vi "Main.vi"(10 "Communication":refnum<class "Communication.lvclass">, 11 "Module Admin":refnum<class "Delacor_lib_QMH_Cloneable Module Admin.lvclass">) -> ()   [LabVIEW 2021, in "Communication.lvlib"]
doc: "This template is based off of the Queued Message Handler design pattern and the Queued Message Handler project template that ships with LabVIEW.\n\nThe main difference is that the queue is private to this module and communication between modules is performed via Broadcast and Request events.\n\nRequest events are wrapped in public API methods and are handled in the Event Handling Loop (EHL) of this VI. Any module can register for Broadcast events sent by this module. The EHL generates messages based on user interface actions.\n\nThe Message Handling Loop (MHL) processes messages generated by the EHL, or by other messages. The messages are string values, so new messages can be added easily to the Message Cases case structure in the MHL. Each message cluster can also provide an optional value for Message Data, which is a variant that can be converted to whatever message-specific data is required.\n_____\nBased on DQMH Dev Tools: Project Template 7.1.2.1547."
uses:
  Communication.lvlib
  <vilib>/Delacor/Delacor QMH/Libraries/Cloneable Module Admin_class/Delacor_lib_QMH_Cloneable Module Admin.lvclass
  C:/Program Files (x86)/National Instruments/LabVIEW 2021/vi.lib/Delacor/Delacor QMH/Libraries/Module Admin_class/Delacor_lib_QMH_Module Admin.lvclass
  Communication/Communication.lvclass
  Module Data--cluster.ctl
  <vilib>/Delacor/Delacor QMH/Libraries/Message Queue_class/Delacor_lib_QMH_Message Queue.lvclass/Delacor_lib_QMH_Message Queue.ctl
  <vilib>/Delacor/Delacor QMH/Libraries/Cloneable Module Admin_class/Delacor_lib_QMH_Cloneable Module Admin.lvclass/Delacor_lib_QMH_Cloneable Module Admin.ctl
  Stop Argument--cluster.ctl
  <vilib>/Delacor/Delacor QMH/Libraries/Module Admin_class/Delacor_lib_QMH_Module Admin.lvclass/Delacor_lib_QMH_Module Admin.ctl
  Show config values Argument--cluster.ctl
  Show config values (Reply Payload)--cluster.ctl
  <vilib>/Utility/miscctls.llb/LVPointTypeDef.ctl
  Communication/Communication.lvclass/Communication.ctl
  <vilib>/Delacor/Delacor QMH/Libraries/Message Queue_class/Delacor_lib_QMH_Enqueue Message (Single).vi
  <vilib>/Delacor/Delacor QMH/Libraries/Cloneable Module Admin_class/Delacor_lib_QMH_Get Module ID.vi
  <vilib>/Delacor/Delacor QMH/Libraries/Module Admin_class/Delacor_lib_QMH_Get External Launch.vi
  <vilib>/Delacor/Delacor QMH/Libraries/Message Queue_class/Delacor_lib_QMH_Message Queue.lvclass
panel:
  out "error out":errorcluster
  out "Status":string
  in  "Simulate EHL Error":bool
  in  "Simulate MHL Error":bool
  # "Other processes communicate with this Module via its Public API (wrappers for its Request Events).\n\nThis Module communicates with other processes via its Broadcast Events.\nAny process that wants to receive these messages can register for this module's Broadcast events."
  # "This template is for the DQMH framework. See the block diagram for more information on how to use this template."
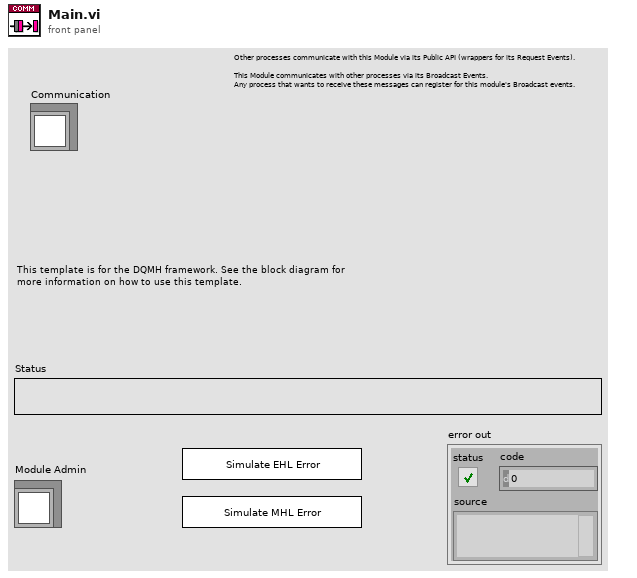
[diagram p1: front panel]
types:
  T1 = typedef "Communication.lvlib/Request Events--cluster.ctl" = cluster{"Stop Module":refnum<user-event>, "Show Panel":refnum<user-event>, "Hide Panel":refnum<user-event>, "Show Diagram":refnum<user-event>, "Get Module Execution Status":refnum<user-event>, "Show config values":refnum<user-event>}
  T2 = typedef "Communication.lvlib/Module Data--cluster.ctl" = cluster{"Status":string}
  T3 = enum32{"invalid lock state", "Not Locked", "Locked (No Password)", "Password-protected"}
  T4 = typedef "Communication.lvlib/Stop Argument--cluster.ctl" = cluster{"Module ID":i32, "Origin":string, "Exit via Stop Module Req?":bool, "Wait for Module to stop?":bool}
  T5 = typedef "Communication.lvlib/Show config values Argument--cluster.ctl" = cluster{"Module ID":i32, "Wait Notifier":refnum<notifier>, "wait for reply":bool}
  T6 = typedef "LVPointTypeDef.ctl" = cluster{"Horizontal":i16, "Vertical":i16}
  T7 = enum32{"Invalid", "Standard", "Closed", "Hidden", "Minimized", "Maximized"}
  T8 = typedef "Communication.lvlib/Show config values (Reply Payload)--cluster.ctl" = cluster{"Module ID":i32, "Comm":cluster{"Path":path}, "error":errorcluster, "params":cluster{"connection_type":string, "baud_rate":i32, "port":string, "Name":string, "ShowFP":bool}}
  T9 = cluster{"connection_type":string, "baud_rate":i32, "port":string, "Name":string, "ShowFP":bool}
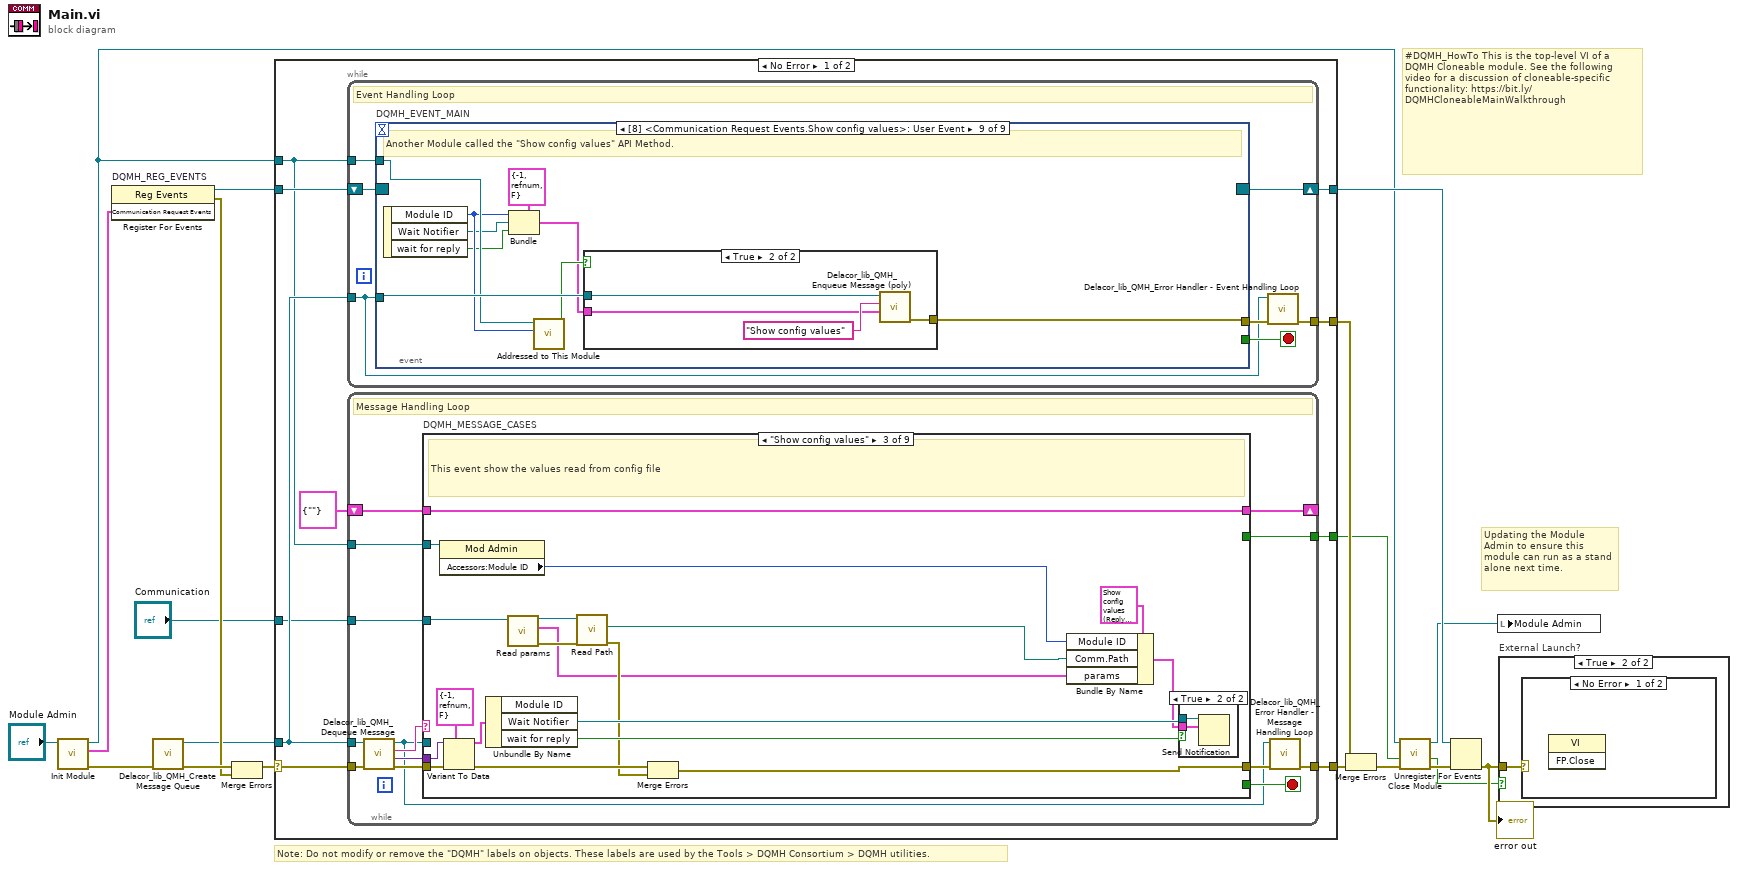
[diagram p0: block diagram]
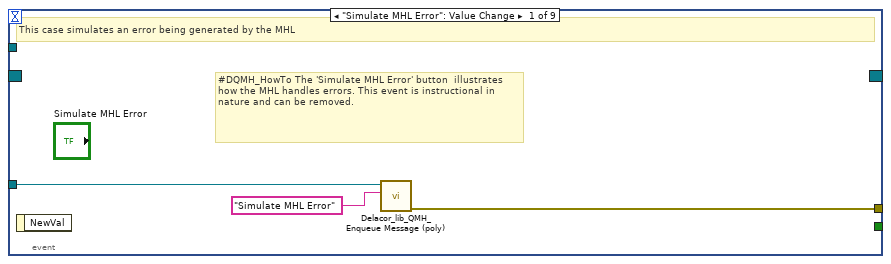
[diagram p2: hidden frame]
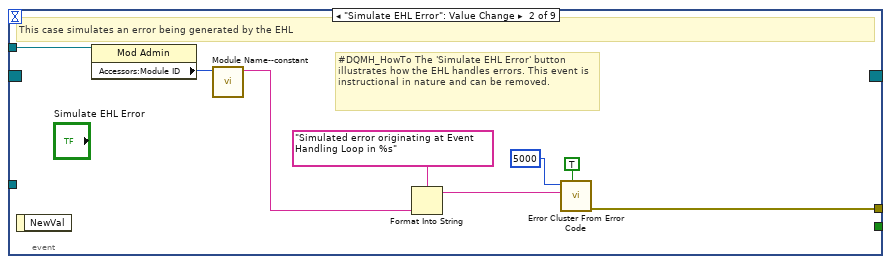
[diagram p3: hidden frame]
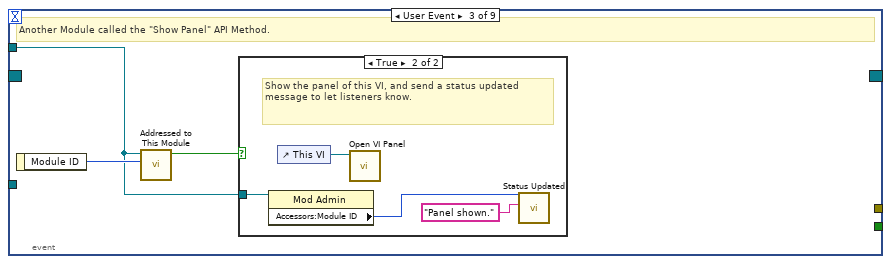
[diagram p4: hidden frame]
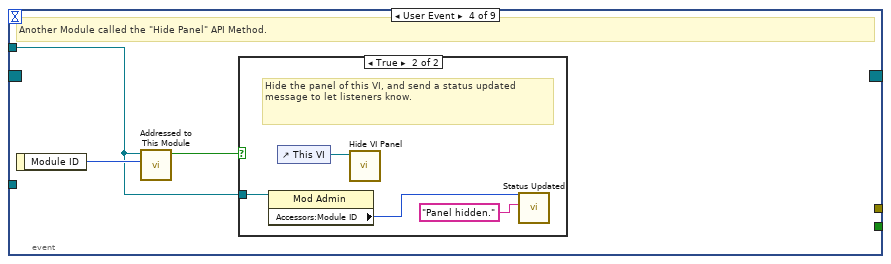
[diagram p6: hidden frame]
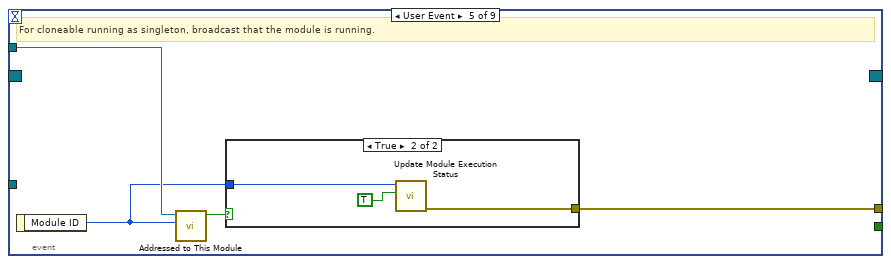
[diagram p8: hidden frame]
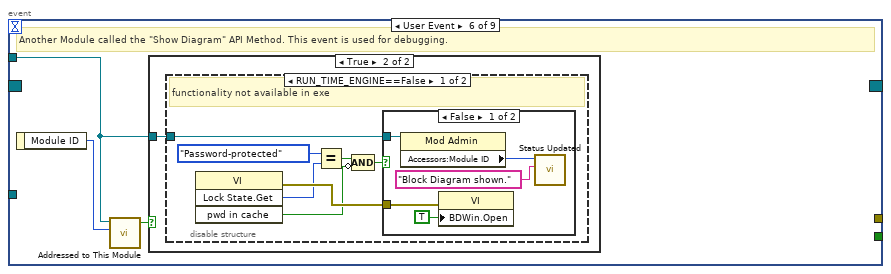
[diagram p10: hidden frame]
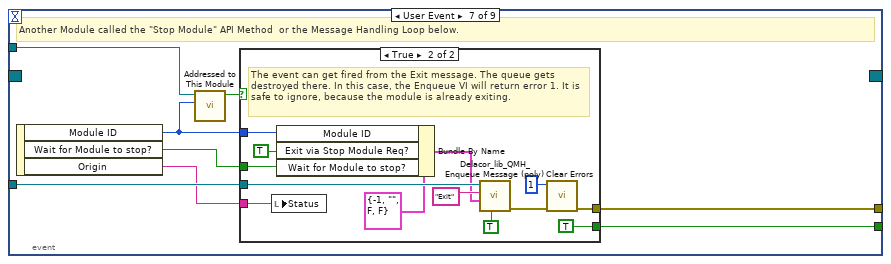
[diagram p14: hidden frame]
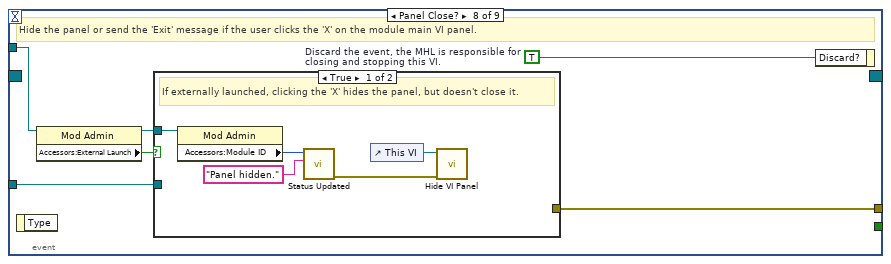
[diagram p16: hidden frame]
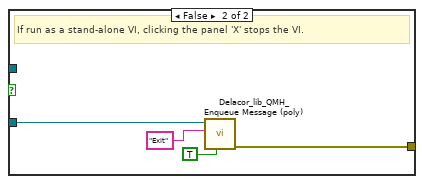
[diagram p17: hidden frame]
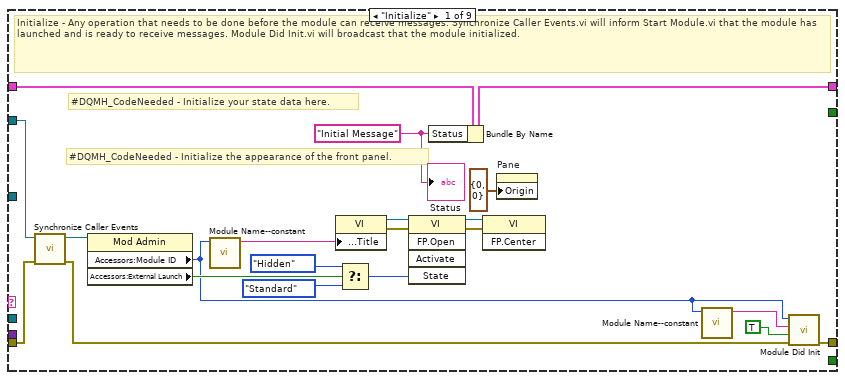
[diagram p19: hidden frame]
diagram:
  # "#DQMH_HowTo This is the top-level VI of a DQMH Cloneable module. See the following video for a discussion of cloneable-specific functionality: https://bit.ly/DQMHCloneableMainWalkthrough"
  # "Note: Do not modify or remove the \"DQMH\" labels on objects. These labels are used by the Tools > DQMH Consortium > DQMH utilities."
  # "Updating the Module Admin to ensure this module can run as a stand alone next time."
  n1 = call "Init Module.vi"("Cloneable Module Admin in"="Module Admin") -> ("error out"=w16:errorcluster, "Communication Request Events"=w8:T1, "Cloneable Module Admin out"=w5:refnum<class "Delacor_lib_QMH_Cloneable Module Admin.lvclass">)  [unwired: 8 in]
  n2 = register-events "DQMH_REG_EVENTS"(w8) -> (reference out=w9:refnum<event-registration>, error out=w11:errorcluster)  [unwired: 2 in]
  n3 = call <vilib>:"Delacor_lib_QMH_Create Message Queue.vi"("error in"=w16) -> ("error out"=w13:errorcluster, "Message Queue"=w7:refnum<class "Delacor_lib_QMH_Message Queue.lvclass">)  [unwired: 9 in]
  n4 = Merge Errors(w13, w11) -> (w12:errorcluster)
  n5 = case shown="No Error" w12 {
    selector: w12 -> [w27 w264]
    tunnel: [w29 w263] -> w17
    tunnel: [w26 w262] -> w10
    tunnel: w9 -> [w24 w262]
    tunnel: w7 -> [w23 w255]
    tunnel: [w28 _] -> w18
    tunnel: w5 -> [w22 w258]
    tunnel: [w21 _] -> w3
    tunnel: "Communication" -> [w20 _]
    frame No Error {
      n6 = while {
        tunnel: w23 -> [w30]
        shift-right: [w33] -> w26
        shift-left: w24 -> [w34]
        tunnel: [w35] -> w28
        tunnel: w22 -> [w31]
        stop <- w32 stop-if-true
        # "Event Handling Loop"
        n7 = event "DQMH_EVENT_MAIN" shown="[8] <Communication Request Events.Show config values>: User Event" {
          selector: w34 -> [_ _ _ _ _ _ _ _ _]
          dyn-events: [_ _ _ _ _ _ _ _ _] -> w33
          timeout: _ -> [_ _ _ _ _ _ _ _ _]
          tunnel: [_ _ _ _ _ _ w88 _ _] -> w32
          tunnel: w30 -> [w38 _ _ _ _ _ w91 w108 w129]
          tunnel: [w39 w47 _ _ w65 _ w92 w111 w121] -> w36
          tunnel: w31 -> [_ w46 w48 w55 w63 w69 w90 w109 w127]
          event "Simulate MHL Error": Value Change {
            # "#DQMH_HowTo The 'Simulate MHL Error' button  illustrates how the MHL handles errors. This event is instructional in nature and can be removed."
            # "This case simulates an error being generated by the MHL"
            n8 = event-data() -> ()  [unwired: 1 in, 1 out]
            n9 = call-poly <vilib>:"Delacor_lib_QMH_Enqueue Message (poly).vi"("Message"="Simulate MHL Error", "Message Queue in"=w38) -> ("error out"=w39:errorcluster)  [unwired: 8 in, 1 out]
          }
          event "Simulate EHL Error": Value Change {
            # "#DQMH_HowTo The 'Simulate EHL Error' button  illustrates how the EHL handles errors. This event is instructional in nature and can be removed."
            # "This case simulates an error being generated by the EHL"
            n10 = event-data() -> ()  [unwired: 1 in, 1 out]
            n11 = property on="Property Node" class="Mod Admin"(reference=w46) -> ("Accessors:Module ID"=w45:i32)  [unwired: 1 in, 2 out]
            n12 = call "Module Name--constant.vi"("Module ID"=w45) -> ("Module Name"=w40:string)  [unwired: 10 in]
            n13 = Format Into String(format string="Simulated error originating at Event Handling Loop in %s", w40) -> (resulting string=w43:string)  [unwired: 2 in, 1 out]
            n14 = call <vilib>:"Error Cluster From Error Code.vi"("show call chain? (False)"=TRUE, "error message (\"\")"=w43, "error code (0)"=5000) -> ("error out"=w47:errorcluster)  [unwired: 6 in]
          }
          event User Event {
            # "Another Module called the \"Show Panel\" API Method."
            n15 = event-data() -> ("Module ID"=w49:i32)  [unwired: 1 in]
            n16 = call "Addressed to This Module.vi"("Module ID from Argument"=w49, "Module Admin"=w48) -> ("Addressed to this instance?"=w50:bool)  [unwired: 8 in, 1 out]
            n17 = case shown="True" w50 {
              tunnel: w48 -> [_ w52]
              frame False {
              }
              frame True {
                # "Show the panel of this VI, and send a status updated message to let listeners know."
                n18 = property on="Property Node" class="Mod Admin"(reference=w52) -> ("Accessors:Module ID"=w51:i32)  [unwired: 1 in, 2 out]
                n19 = control-ref of="This VI"() -> (w54:refnum<vi>)
                n20 = call "Open VI Panel.vi"("VI"=w54) -> ()  [unwired: 10 in, 1 out]
                n21 = call "Status Updated.vi"("Status"="Panel shown." ("format string"), "Module ID"=w51) -> ()  [unwired: 9 in, 1 out]
              }
            }
          }
          event User Event {
            # "Another Module called the \"Hide Panel\" API Method."
            n22 = event-data() -> ("Module ID"=w56:i32)  [unwired: 1 in]
            n23 = call "Addressed to This Module.vi"("Module ID from Argument"=w56, "Module Admin"=w55) -> ("Addressed to this instance?"=w57:bool)  [unwired: 8 in, 1 out]
            n24 = case shown="True" w57 {
              tunnel: w55 -> [_ w59]
              frame False {
              }
              frame True {
                # "Hide the panel of this VI, and send a status updated message to let listeners know."
                n25 = property on="Property Node" class="Mod Admin"(reference=w59) -> ("Accessors:Module ID"=w58:i32)  [unwired: 1 in, 2 out]
                n26 = control-ref of="This VI"() -> (w61:refnum<vi>)
                n27 = call "Hide VI Panel.vi"("VI"=w61) -> ()  [unwired: 10 in, 1 out]
                n28 = call "Status Updated.vi"("Status"="Panel hidden." ("format string"), "Module ID"=w58) -> ()  [unwired: 9 in, 1 out]
              }
            }
          }
          event User Event {
            # "For cloneable running as singleton, broadcast that the module is running."
            n29 = event-data() -> ("Module ID"=w62:i32)  [unwired: 1 in]
            n30 = call "Addressed to This Module.vi"("Module ID from Argument"=w62, "Module Admin"=w63) -> ("Addressed to this instance?"=w64:bool)  [unwired: 8 in, 1 out]
            n31 = case shown="True" w64 {
              tunnel: [_ w68] -> w65
              tunnel: w62 -> [_ w67]
              frame False {
              }
              frame True {
                n32 = call "Update Module Execution Status.vi"("Running?"=TRUE, "Module ID"=w67) -> ("error out"=w68:errorcluster)  [unwired: 9 in]
              }
            }
          }
          event User Event {
            # "Another Module called the \"Show Diagram\" API Method. This event is used for debugging."
            n33 = event-data() -> ("Module ID"=w70:i32)  [unwired: 1 in]
            n34 = call "Addressed to This Module.vi"("Module ID from Argument"=w70, "Module Admin"=w69) -> ("Addressed to this instance?"=w71:bool)  [unwired: 8 in, 1 out]
            n35 = case shown="True" w71 {
              tunnel: w69 -> [_ w72]
              frame False {
              }
              frame True {
                n36 = disable-structure shown="RUN_TIME_ENGINE==False" {
                  disable-tunnel: w72 -> [w73 _]
                  frame condition #0 (active) {
                    # "functionality not available in exe"
                    n37 = invoke on="Invoke Node" class="VI" method="Lock State.Get"() -> (error out=w79:errorcluster, "Get Lock State"=w78:T3, "pwd in cache"=w75:bool)  [unwired: 4 in, 1 out]
                    n38 = Equal?(x=T3."Password-protected", y=w78) -> (x = y?=w76:bool)
                    n39 = Compound Arithmetic op=AND(w76, invert w75) -> (w74:bool)
                    n40 = case shown="False" w74 {
                      tunnel: w79 -> [w84 _]
                      tunnel: w73 -> [w81 _]
                      frame False {
                        n41 = property on="Property Node" class="Mod Admin"(reference=w81) -> ("Accessors:Module ID"=w80:i32)  [unwired: 1 in, 2 out]
                        n42 = property on="Property Node" class="VI"(error in=w84, "BDWin.Open"=TRUE ("Block Diagram Window:Open")) -> ()  [unwired: 1 in, 2 out]
                        n43 = call "Status Updated.vi"("Status"="Block Diagram shown." ("format string"), "Module ID"=w80) -> ()  [unwired: 9 in, 1 out]
                      }
                      frame True {
                        # "Password-protected VI, and the password is not in the cache. Do not show the diagram."
                      }
                    }
                  }
                  frame condition #1 {
                  }
                }
              }
            }
          }
          event User Event {
            # "Another Module called the \"Stop Module\" API Method  or the Message Handling Loop below."
            n44 = event-data() -> ("Module ID"=w86:i32, "Wait for Module to stop?"=w87:bool, "Origin"=w85:string)  [unwired: 1 in]
            n45 = call "Addressed to This Module.vi"("Module ID from Argument"=w86, "Module Admin"=w90) -> ("Addressed to this instance?"=w89:bool)  [unwired: 8 in, 1 out]
            n46 = case shown="True" w89 {
              tunnel: [_ w104] -> w92
              tunnel: w91 -> [_ w100]
              tunnel: [_ TRUE] -> w88
              tunnel: w87 -> [_ w95]
              tunnel: w86 -> [_ w97]
              tunnel: w85 -> [_ w93]
              frame False {
              }
              frame True {
                # "The event can get fired from the Exit message. The queue gets destroyed there. In this case, the Enqueue VI will return error 1. It is safe to ignore, because the module is already exiting."
                n47 = local write "Status"(w93) -> ()
                n48 = Bundle By Name(cluster=T4 {"Module ID"=-1, "Origin"="", "Exit via Stop Module Req?"=FALSE, "Wait for Module to stop?"=FALSE} ("Stop Argument"), "Module ID"=w97, "Exit via Stop Module Req?"=TRUE, "Wait for Module to stop?"=w95) -> (w94:T4)
                n49 = call-poly <vilib>:"Delacor_lib_QMH_Enqueue Message (poly).vi"("Priority Message? (F)"=TRUE, "Message Data"=w94, "Message"="Exit", "Message Queue in"=w100) -> ("error out"=w105:errorcluster)  [unwired: 6 in, 1 out]
                n50 = call <vilib>:"Clear Errors.vi"("error in (no error)"=w105, "specific error code to clear (0: all)"=1) -> ("error out"=w104:errorcluster)  [unwired: 4 in, 1 out]
              }
            }
          }
          event Panel Close? {
            w110 = TRUE  # Discard the event, the MHL is responsible for closing and stopping this VI.
            # "Hide the panel or send the 'Exit' message if the user clicks the 'X' on the module main VI panel."
            n51 = event-data() -> ()  [unwired: 1 in, 1 out]
            n52 = property on="Property Node" class="Mod Admin"(reference=w109) -> (reference out=w106:refnum<class "Delacor_lib_QMH_Cloneable Module Admin.lvclass">, "Accessors:External Launch"=w107:bool)  [unwired: 1 in, 1 out]
            n53 = case shown="True" w107 {
              tunnel: w108 -> [_ w119]
              tunnel: [_ w120] -> w111
              tunnel: w106 -> [w114 _]
              frame True {
                # "If externally launched, clicking the 'X' hides the panel, but doesn't close it."
                n54 = property on="Property Node" class="Mod Admin"(reference=w114) -> ("Accessors:Module ID"=w113:i32)  [unwired: 1 in, 2 out]
                n55 = call "Status Updated.vi"("Status"="Panel hidden." ("format string"), "Module ID"=w113) -> ("error out"=w112:errorcluster)  [unwired: 9 in]
                n56 = control-ref of="This VI"() -> (w116:refnum<vi>)
                n57 = call "Hide VI Panel.vi"("error in"=w112, "VI"=w116) -> ()  [unwired: 9 in, 1 out]
              }
              frame False {
                # "If run as a stand-alone VI, clicking the panel 'X' stops the VI."
                n58 = call-poly <vilib>:"Delacor_lib_QMH_Enqueue Message (poly).vi"("Priority Message? (F)"=TRUE, "Message"="Exit", "Message Queue in"=w119) -> ("error out"=w120:errorcluster)  [unwired: 7 in, 1 out]
              }
            }
            n59 = event-data ("Event Filter Node")("Discard?"=w110) -> ()  [unwired: 1 in, 1 out]
          }
          event User Event {
            # "Another Module called the \"Show config values\" API Method."
            n60 = event-data() -> ("Module ID"=w124:i32, "Wait Notifier"=w123:refnum<notifier>, "wait for reply"=w122:bool)  [unwired: 1 in]
            n61 = Bundle(cluster=T5 {"Module ID"=-1, "Wait Notifier"=refnum, "wait for reply"=FALSE} ("Show config values Argument"), "Module ID"=w124, "Wait Notifier"=w123, "wait for reply"=w122) -> (w125:T5)
            n62 = call "Addressed to This Module.vi"("Module ID from Argument"=w124, "Module Admin"=w127) -> ("Addressed to this instance?"=w128:bool)  [unwired: 8 in, 1 out]
            n63 = case shown="True" w128 {
              tunnel: w129 -> [_ w133]
              tunnel: w125 -> [_ w131]
              tunnel: [_ w130] -> w121
              frame False {
              }
              frame True {
                n64 = call-poly <vilib>:"Delacor_lib_QMH_Enqueue Message (poly).vi"("Message Data"=w131, "Message"="Show config values", "Message Queue in"=w133) -> ("error out"=w130:errorcluster)  [unwired: 7 in, 1 out]
              }
            }
          }
        }
        n65 = call-dynamic "Delacor_lib_QMH_Error Handler - Event Handling Loop.vi"("error in"=w36, "Message Queue in"=w30) -> ("dup error in"=w35:errorcluster)  [unwired: 8 in, 1 out]
      }
      n66 = while {
        tunnel: w23 -> [w135]
        shift-right: [w142] -> _
        shift-left: T2 {"Status"=""} ("Data Cluster") -> [w143]
        tunnel: w27 -> [w146]
        tunnel: [w144] -> w29
        tunnel: w22 -> [w137]
        tunnel: [w136] -> w21
        tunnel: w20 -> [w134]
        stop <- w141 stop-if-true
        # "Message Handling Loop"
        n67 = call-dynamic "Delacor_lib_QMH_Dequeue Message.vi"("error in"=w146, "Message Queue in"=w135) -> ("error out"=w145:errorcluster, "Message Data"=w139:variant, "Message"=w140:string, "Message Queue out"=w138:refnum<class "Delacor_lib_QMH_Message Queue.lvclass">)  [unwired: 6 in]
        n68 = case "DQMH_MESSAGE_CASES" shown="\"Show config values\"" w140 {
          selector: w140 -> [_ _ _ _ _ _ _ _ w244]
          tunnel: w138 -> [_ _ _ _ _ w199 _ w236 _]
          tunnel: w145 -> [w166 w170 w189 w194 w196 w208 w225 w242 w253]
          tunnel: [w164 w170 w179 w193 w196 w204 w224 w237 w254] -> w147
          tunnel: w143 -> [w157 w169 w188 w192 w195 w203 w222 w235 w251]
          tunnel: [w156 w169 w188 w192 w195 w203 w222 w235 w251] -> w142
          tunnel: [_ _ _ _ _ _ _ w234 _] -> w141
          tunnel: w139 -> [_ _ w186 _ _ w202 _ w232 _]
          tunnel: w137 -> [w152 _ w177 _ _ w201 w220 w227 w250]
          tunnel: [_ _ _ _ _ _ _ w230 _] -> w136
          tunnel: w134 -> [_ _ w173 _ _ _ _ _ _]
          frame "Initialize" {
            w149 = "Initial Message" ("Initial Message")
            # "#DQMH_CodeNeeded - Initialize the appearance of the front panel."
            # "#DQMH_CodeNeeded - Initialize your state data here."
            # "Initialize - Any operation that needs to be done before the module can receive messages. Synchronize Caller Events.vi will inform Start Module.vi that the module has launched and is ready to receive messages. Module Did Init.vi will broadcast that the module initialized."
            n69 = call "Synchronize Caller Events.vi"("error in"=w166, "Module Admin"=w152) -> ("error out"=w165:errorcluster, "Module Admin out"=w151:refnum<class "Delacor_lib_QMH_Cloneable Module Admin.lvclass">)  [unwired: 8 in]
            n70 = property on="Property Node" class="Mod Admin"(reference=w151) -> ("Accessors:Module ID"=w148:i32, "Accessors:External Launch"=w153:bool)  [unwired: 1 in, 2 out]
            n71 = call "Module Name--constant.vi"("Module ID"=w148) -> ("Module Name"=w161:string)  [unwired: 10 in]
            n72 = property on="Property Node" class="VI"("Front Panel.Title"=w161) -> (reference out=w163:refnum<vi>, error out=w168:errorcluster)  [unwired: 2 in]
            n73 = Select(t=T7."Hidden" ("State"), s=w153, f=T7."Standard" ("State")) -> (s? t:f=w158:T7)
            n74 = invoke on="Invoke Node" class="VI" method="FP.Open"(reference=w163, error in=w168, "State"=w158) -> (reference out=w162:refnum<vi>, error out=w167:errorcluster)  [unwired: 2 in, 3 out]
            n75 = Bundle By Name(cluster=w157, "Status"=w149) -> (w156:T2)
            n76 = invoke on="Invoke Node" class="VI" method="FP.Center"(reference=w162, error in=w167) -> ()  [unwired: 1 in, 3 out]
            n77 = property on="Pane" class="Pane"("Origin"=T6 {"Horizontal"=0, "Vertical"=0}) -> ()  [unwired: 2 in, 2 out]
            n78 = call "Module Name--constant.vi"("Module ID"=w148) -> ("Module Name"=w154:string)  [unwired: 10 in]
            n79 = call "Module Did Init.vi"("error in"=w165, "Initialized?"=TRUE, "Origin"=w154, "Module ID"=w148) -> ("error out"=w164:errorcluster)  [unwired: 7 in]
            "Status" <- w149
          }
          frame "---Module Specific---" {
            # "Separator -- The following cases handle messages specific to this Module."
          }
          frame "Show config values" {
            # "This event show the values read from config file"
            n80 = property class="Mod Admin"(reference=w177) -> ("Accessors:Module ID"=w178:i32)  [unwired: 1 in, 2 out]
            n81 = Variant To Data(error in=w189, type=T5 {"Module ID"=-1, "Wait Notifier"=refnum, "wait for reply"=FALSE} ("Show config values Argument"), Variant=w186) -> (data=w184:T5, error out=w187:errorcluster)
            n82 = Unbundle By Name(w184) -> ("Wait Notifier"=w183:refnum<notifier>, "wait for reply"=w182:bool)  [unwired: 1 out]
            n83 = call "Read params.vi"("Communication in"=w173) -> ("error out"=w174:errorcluster, "params"=w171:T9, "Communication out"=w175:refnum<class "Communication.lvclass">)  [unwired: 8 in]
            n84 = call "Read Path.vi"("error in (no error)"=w174, "Communication in"=w175) -> ("error out"=w172:errorcluster, "Path"=w176:path)  [unwired: 7 in, 1 out]
            n85 = Merge Errors(w187, w172) -> (w179:errorcluster)
            n86 = Bundle By Name(cluster=T8 {"Module ID"=-1, "Comm"={"Path"=path ""}, "error"={"status"=FALSE, "code"=0, "source"=""}, "params"={"connection_type"="", "baud_rate"=0, "port"="", "Name"="", "ShowFP"=FALSE}} ("Show config values (Reply Payload)"), "Module ID"=w178, "Comm.Path"=w176, "params"=w171) -> (w181:T8)
            n87 = case "DQMH_FIRE_NOTIFIER" shown="True" w182 {
              tunnel: w183 -> [_ w191]
              tunnel: w181 -> [_ w190]
              frame False {
              }
              frame True {
                n88 = Send Notification(notification=w190, notifier=w191) -> ()  [unwired: 1 in, 2 out]
              }
            }
          }
          frame "---Copy This Frame---" {
            # "Duplicate this frame when creating new messages.  Change this comment in the duplicated frame to describe this message."
            n89 = Merge Errors(w194) -> (w193:errorcluster)
          }
          frame "---Exit and Error Handling---" {
            # "Separator - the following cases handle errors and exit messages."
          }
          frame "Error" {
            # "#DQMH_CodeRecommended - If the module is running in standalone mode (External Launch = FALSE), this code will pop up an error dialog and call the 'Exit' message if an error occurs. Add more fine-grained error management here."
            # "Error - Check the error message data and respond accordingly. This message is sent by the \"Error Handler\" VIs at the end of each loop in this application."
            n90 = property on="Property Node" class="Mod Admin"(reference=w201) -> ("Accessors:External Launch"=w200:bool, "Accessors:Module ID"=w198:i32)  [unwired: 1 in, 2 out]
            n91 = Variant To Data(error in=w208, type=errorcluster {"status"=FALSE, "code"=0, "source"=""} ("error constant"), Variant=w202) -> (data=w197:errorcluster, error out=w206:errorcluster)
            n92 = local write "error out"(w197) -> ()
            n93 = call "Error Reported.vi"("Error"=w197, "Module ID"=w198) -> ()  [unwired: 9 in, 1 out]
            n94 = case shown="False" w200 {
              tunnel: [w213 _] -> w205
              tunnel: w199 -> [w211 _]
              tunnel: w197 -> [w212 _]
              frame False {
                n95 = disable-structure shown="Default" {
                  disable-tunnel: w212 -> [w214 _]
                  frame condition #0 (active) {
                    # "If the module is running standalone, then pop up an error dialog and call the \"Exit\" message."
                    n96 = call <vilib>:"Simple Error Handler.vi"("error in (no error)"=w214) -> ()  [unwired: 4 in, 5 out]
                  }
                  frame condition #1 {
                    # "To prevent the Simple Error Handler VI from being loaded (e.g. when deploying to a Real-Time target), add the Conditional Disable Symbol \"DQMH_Disable_SEH\" to your project and set it to TRUE."
                  }
                }
                n97 = call-poly <vilib>:"Delacor_lib_QMH_Enqueue Message (poly).vi"("Priority Message? (F)"=TRUE, "Message"="Exit", "Message Queue in"=w211) -> ("error out"=w213:errorcluster)  [unwired: 7 in, 1 out]
              }
              frame True {
                # "If the module was launched externally, calling the Error Reported broadcast VI is the only action performed by the \"Error\" message. The module's caller can then process the error appropriately."
              }
            }
            n98 = Merge Errors(w206, w205) -> (w204:errorcluster)
          }
          frame "Simulate MHL Error" {
            # "#DQMH_HowTo The 'Simulate MHL Error' button  illustrates how the MHL handles errors. This event is instructional in nature and can be removed."
            # "Simulate an error occurring at the MHL"
            n99 = property on="Property Node" class="Mod Admin"(reference=w220) -> ("Accessors:Module ID"=w221:i32)  [unwired: 1 in, 2 out]
            n100 = call "Module Name--constant.vi"("Module ID"=w221) -> ("Module Name"=w216:string)  [unwired: 10 in]
            n101 = Format Into String(format string="Simulated error originating at Message Handling Loop in %s", w216) -> (resulting string=w217:string)  [unwired: 2 in, 1 out]
            n102 = call <vilib>:"Error Cluster From Error Code.vi"("show call chain? (False)"=TRUE, "error message (\"\")"=w217, "error code (0)"=5001) -> ("error out"=w223:errorcluster)  [unwired: 6 in]
            n103 = Merge Errors(w225, w223) -> (w224:errorcluster)
          }
          frame "Exit" {
            w233 = 91  # 91: not all Exit messages will have an argument
            w234 = TRUE  # Stop the VI
            # "Release the message queue reference"
            # "#DQMH_CodeNeeded - Add any required cleanup code here."
            # "Exit - Exit the application."
            n104 = Variant To Data(error in=w242, type=T4 {"Module ID"=-1, "Origin"="", "Exit via Stop Module Req?"=FALSE, "Wait for Module to stop?"=FALSE} ("Stop Argument"), Variant=w232) -> (data=w229:T4, error out=w238:errorcluster)
            n105 = call <vilib>:"Clear Errors.vi"("error in (no error)"=w238, "specific error code to clear (0: all)"=w233) -> ("error out"=w241:errorcluster)  [unwired: 4 in, 1 out]
            n106 = property on="Property Node" class="Mod Admin"(reference=w227) -> ("Accessors:Module ID"=w226:i32)  [unwired: 1 in, 2 out]
            n107 = control-ref of="This VI"() -> (w228:refnum<vi>)
            n108 = call-dynamic "Delacor_lib_QMH_Release Message Queue.vi"("error in"=w241, "Message Queue"=w236) -> ("error out"=w240:errorcluster)  [unwired: 9 in]
            n109 = call "Handle Exit.vi"("Stop Argument"=w229, "Module Admin in"=w227, "VI reference"=w228) -> ("error out"=w239:errorcluster, "Wait for Stop?"=w230:bool)  [unwired: 7 in]
            n110 = Merge Errors(w240, w239) -> (w237:errorcluster)
            n111 = call "Error Reported.vi"("Error"=w237, "Module ID"=w226) -> ()  [unwired: 9 in, 1 out]
          }
          frame Default {
            # "'Default' case only runs if there is a message that isn't defined in any of the other cases.  Output a programming error."
            n112 = property on="Property Node" class="Mod Admin"(reference=w250) -> ("Accessors:Module ID"=w249:i32)  [unwired: 1 in, 2 out]
            n113 = call "Module Name--constant.vi"("Module ID"=w249) -> ("Module Name"=w243:string)  [unwired: 10 in]
            n114 = Format Into String(format string="The invalid message string \"%s\" was received in the Message Handling Loop for module \"%s\".", w244, w243) -> (resulting string=w246:string)  [unwired: 2 in, 1 out]
            n115 = call <vilib>:"Error Cluster From Error Code.vi"("show call chain? (False)"=TRUE, "error message (\"\")"=w246, "error code (0)"=1) -> ("error out"=w252:errorcluster)  [unwired: 6 in]
            n116 = Merge Errors(w253, w252) -> (w254:errorcluster)
          }
        }
        n117 = call-dynamic "Delacor_lib_QMH_Error Handler - Message Handling Loop.vi"("error in"=w147, "Message Queue in"=w138) -> ("dup error in"=w144:errorcluster)  [unwired: 8 in, 1 out]
      }
    }
    frame Error {
      n118 = call "Synchronize Caller Events.vi"("Module Admin"=w258) -> ("Module Admin out"=w257:refnum<class "Delacor_lib_QMH_Cloneable Module Admin.lvclass">)  [unwired: 9 in, 1 out]
      n119 = property on="Property Node" class="Mod Admin"(reference=w257) -> ("Accessors:Module ID"=w256:i32)  [unwired: 1 in, 2 out]
      n120 = call-dynamic "Delacor_lib_QMH_Release Message Queue.vi"("error in"=w264, "Message Queue"=w255) -> ("error out"=w263:errorcluster)  [unwired: 9 in]
      n121 = call "Module Name--constant.vi"("Module ID"=w256) -> ("Module Name"=w261:string)  [unwired: 10 in]
      n122 = Format Into String(format string="An error occurred during initialization. %s is no longer running.", w261) -> (resulting string=w259:string)  [unwired: 2 in, 1 out]
      n123 = call "Error Reported.vi"("Additional Information"=w259, "Error"=w263, "Module ID"=w256) -> ()  [unwired: 8 in, 1 out]
    }
  }
  n124 = Merge Errors(w18, w17) -> (w19:errorcluster)
  n125 = call "Close Module.vi"("error in"=w19, "Wait for stop?"=w3, "Module Admin in"=w5) -> ("error out"=w15:errorcluster, "External Launch"=w2:bool, "Module Admin out"=w4:refnum<class "Delacor_lib_QMH_Cloneable Module Admin.lvclass">)  [unwired: 6 in]
  n126 = Unregister For Events(event registration refnum=w10, error in=w15) -> (error out=w14:errorcluster)
  "error out" <- w14
  n127 = local write "Module Admin"(w4) -> ()
  n128 = case "External Launch?" shown="True" w2 {
    tunnel: w14 -> [_ w265]
    frame False {
    }
    frame True {
      n129 = case shown="No Error" w265 {
        frame No Error {
          n130 = invoke class="VI" method="FP.Close"() -> ()  [unwired: 3 in, 3 out]
        }
        frame Error {
          n131 = disable-structure shown="Default" {
            frame condition #0 (active) {
              n132 = invoke class="VI" method="FP.Open"("Activate"=TRUE ("Activate?")) -> ()  [unwired: 4 in, 5 out]
            }
            frame condition #1 {
              # "Don't show panel on error if running inside a built EXE."
            }
          }
        }
      }
    }
  }
